vi "Get IConfiguration.vi"(11 "PCAN-USB Read-Write Raw CAN Frame Strategy in":refnum<class "PCAN Base Strategy.lvclass">) -> (2 "IConfiguration":refnum<class "IConfiguration.lvclass">, 3 "PCAN-USB Read-Write Raw CAN Frame Strategy out":refnum<class "PCAN Base Strategy.lvclass">)   [LabVIEW 2025, in "PCAN Base Strategy.lvclass"]
uses:
  PCAN Base Strategy.lvclass
  Source/Interfaces/IConfiguration/IConfiguration.lvclass
  PCAN Base Strategy.lvclass/PCAN Base Strategy.ctl
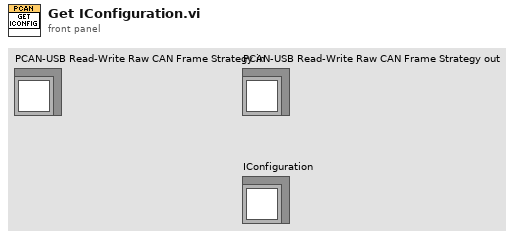
[diagram p1: front panel]
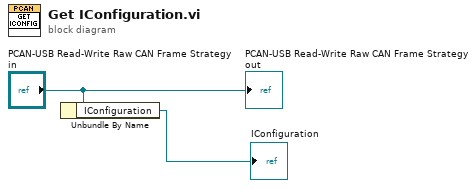
[diagram p0: block diagram]
diagram:
  n1 = Unbundle By Name("PCAN-USB Read-Write Raw CAN Frame Strategy in") -> ("IConfiguration"=→"IConfiguration":refnum<class "IConfiguration.lvclass">)
  "PCAN-USB Read-Write Raw CAN Frame Strategy out" <- "PCAN-USB Read-Write Raw CAN Frame Strategy in"
